vi "Write.vi"(9 "Discrete":bool[](array[boolean]), 11 "TCP Connection Refnum in":refnum<k5>) -> ()   [LabVIEW 2012]
uses:
  MB Ethernet Master Query Folder/NI Modbus.llb/MB Modbus Command.ctl
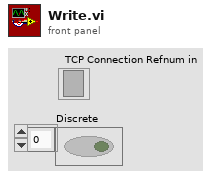
[diagram p1: front panel]
types:
  T1 = typedef "MB Modbus Command.ctl" = cluster{"Function Code":u8, "Starting Address":u16, "Quantity":u16, "Data":u16[], "Discrete":bool[]}
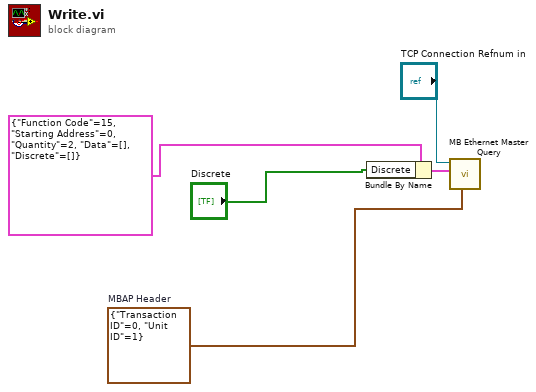
[diagram p0: block diagram]
diagram:
  w4 = cluster{"Transaction ID":u16, "Unit ID":u8} {"Transaction ID"=0, "Unit ID"=1}  # MBAP Header
  n1 = Bundle By Name(cluster=T1 {"Function Code"=15, "Starting Address"=0, "Quantity"=2, "Data"=[], "Discrete"=[]} ("MODBUS Command"), "Discrete"="Discrete") -> (w5:T1)
  n2 = call "MB Ethernet Master Query.vi"("MBAP Header"=w4, "Modbus Command"=w5, "TCP Connection Refnum in"="TCP Connection Refnum in") -> ()  [unwired: 4 in, 5 out]
